vi "S2DS_gmail.vi"(5 "Body":string="It works!", 6 "error in (no error)":errorcluster, 7 "Subject":string="Sending TLS Authenticated Email", 8 "Recipient's Name":string="Jane Doe", 9 "Recipient's Email Address Address":string) -> (0 "error out":errorcluster)   [LabVIEW 2025]
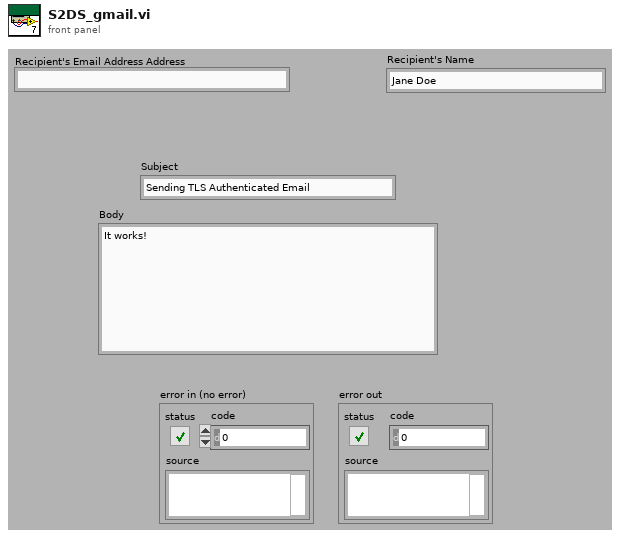
[diagram p1: front panel]
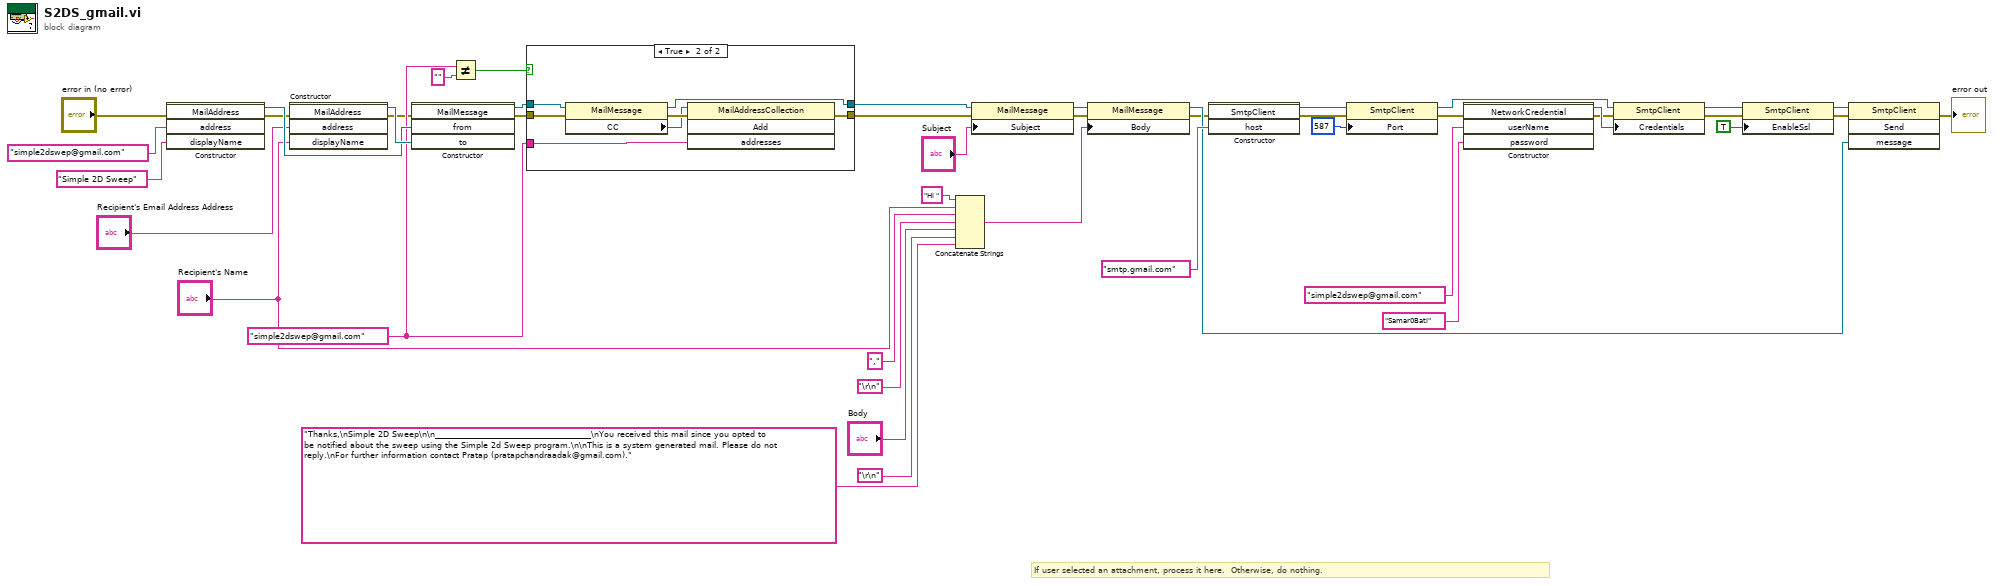
[diagram p0: block diagram]
diagram:
  w21 = "simple2dswep@gmail.com" ("CC (Carbon Copy Recipient - Optional)")
  # "If user selected an attachment, process it here.  Otherwise, do nothing."
  n1 = constructor class="MailAddress"(error in="error in (no error)", "address"="simple2dswep@gmail.com" ("Sender's Email Address (eg: jsmith77@gmail.com)"), "displayName"="Simple 2D Sweep" ("Sender's Name")) -> (reference out=w43:refnum<k24>, error out=w14:errorcluster)  [unwired: 2 in, 3 out]
  n2 = constructor class="MailAddress"(error in=w14, "address"="Recipient's Email Address Address", "displayName"="Recipient's Name") -> (reference out=w44:refnum<k24>, error out=w13:errorcluster)  [unwired: 2 in, 3 out]
  n3 = constructor class="MailMessage"(error in=w13, "from"=w43, "to"=w44) -> (reference out=w20:refnum<k24>, error out=w19:errorcluster)  [unwired: 2 in, 3 out]
  n4 = Not Equal?(x=w21, y="") -> (x != y?=w22:bool)
  n5 = case shown="True" w22 {
    tunnel: w21 -> [_ w51]
    tunnel: w20 -> [w46 w50]
    tunnel: w19 -> [w45 w49]
    tunnel: [w46 w48] -> w18
    tunnel: [w45 w47] -> w17
    frame False {
    }
    frame True {
      n6 = property class="MailMessage"(reference=w50, error in=w49) -> (reference out=w48:refnum<k24>, error out=w53:errorcluster, "CC"=w52:refnum<k24>)
      n7 = invoke class="MailAddressCollection" method="Add"(reference=w52, error in=w53, "addresses"=w51) -> (error out=w47:errorcluster)  [unwired: 1 in, 3 out]
    }
  }
  n8 = Concatenate Strings("Hi " ("string"), "Recipient's Name", "," ("string"), "\r\n", "Body", "\r\n", "Thanks,\nSimple 2D Sweep\n\n_______________________________________\nYou received this mail since you opted to be notified about the sweep using the Simple 2d Sweep program.\n\nThis is a system generated mail. Please do not reply.\nFor further information contact Pratap (pratapchandraadak@gmail.com)." ("string")) -> (w3:string)
  n9 = property class="MailMessage"(reference=w18, error in=w17, "Subject"="Subject") -> (reference out=w36:refnum<k24>, error out=w42:errorcluster)
  n10 = property class="MailMessage"(reference=w36, error in=w42, "Body"=w3) -> (reference out=w16:refnum<k24>, error out=w12:errorcluster)
  n11 = constructor class="SmtpClient"(error in=w12, "host"="smtp.gmail.com" ("Outgoing Mail Server (SMTP)")) -> (reference out=w30:refnum<k24>, error out=w26:errorcluster)  [unwired: 2 in, 2 out]
  n12 = property class="SmtpClient"(reference=w30, error in=w26, "Port"=587) -> (reference out=w29:refnum<k24>, error out=w11:errorcluster)
  n13 = constructor class="NetworkCredential"(error in=w11, "userName"="simple2dswep@gmail.com" ("GMAIL Account User ID (eg: jsmity77)"), "password"="Samar0Bati" ("GMAIL Account Password")) -> (reference out=w31:refnum<k24>, error out=w10:errorcluster)  [unwired: 2 in, 3 out]
  n14 = property class="SmtpClient"(reference=w29, error in=w10, "Credentials"=w31) -> (reference out=w28:refnum<k24>, error out=w25:errorcluster)
  n15 = property class="SmtpClient"(reference=w28, error in=w25, "EnableSsl"=TRUE ("Enable SSL")) -> (reference out=w27:refnum<k24>, error out=w24:errorcluster)
  n16 = invoke class="SmtpClient" method="Send"(reference=w27, error in=w24, "message"=w16) -> (error out=→"error out":errorcluster)  [unwired: 1 in, 3 out]
